vi "Close Active Workspace.vi"(8 "error in (no error)":errorcluster) -> (0 "error out":errorcluster)   [LabVIEW 2014]
uses:
  NationalInstruments.VeriStand.ClientAPI
  <vilib>/NI Veristand/Execution/Project/NI_VS Project ExecutionAPI.lvlib
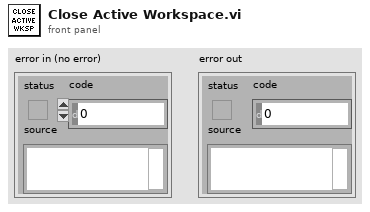
[diagram p1: front panel]
types:
  T1 = typedef "NI_VS Project ExecutionAPI.lvlib/Project Ref.ctl" = refnum<k24>
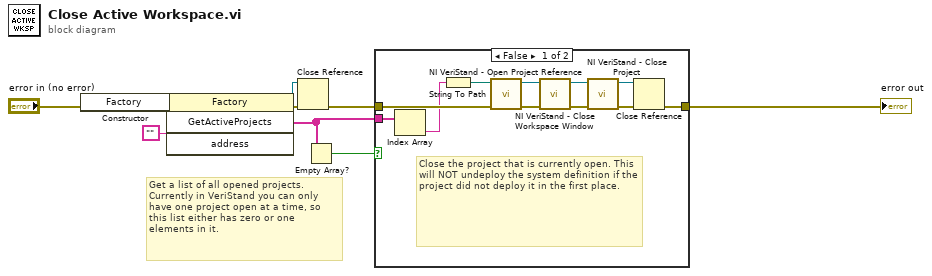
[diagram p0: block diagram]
diagram:
  # "Get a list of all opened projects. Currently in VeriStand you can only have one project open at a time, so this list either has zero or one elements in it."
  n1 = constructor class="Factory"(error in="error in (no error)") -> (reference out=w1:refnum<k24>, error out=w2:errorcluster)  [unwired: 2 in, 1 out]
  n2 = invoke class="Factory" method="GetActiveProjects"(reference=w1, error in=w2, "address"="") -> (reference out=w4:refnum<k24>, error out=w3:errorcluster, "GetActiveProjects"=w7:string[])  [unwired: 1 in, 1 out]
  n3 = Close Reference(reference=w4, error in (no error)=w3) -> (error out=w6:errorcluster)
  n4 = Empty Array?(array=w7) -> (empty?=w8:bool)
  n5 = case shown="False" w8 {
    tunnel: w7 -> [w21 _]
    tunnel: w6 -> [w20 w22]
    tunnel: [w15 w22] -> w9
    frame False {
      # "Close the project that is currently open. This will NOT undeploy the system definition if the project did not deploy it in the first place."
      n6 = Index Array(array=w21) -> (element=w19:string)  [unwired: 1 in]
      n7 = String To Path(string=w19) -> (path=w18:path)
      n8 = call <vilib>:"NI VeriStand - Open Project Reference.vi"("error in (no error)"=w20, "Project File Path"=w18) -> ("error out"=w13:errorcluster, "Project Ref"=w14:T1)  [unwired: 8 in]
      n9 = call <vilib>:"NI VeriStand - Close Workspace Window.vi"("error in (no error)"=w13, "Project Ref in"=w14) -> ("error out"=w12:errorcluster, "Project Ref out"=w11:T1)  [unwired: 8 in]
      n10 = call <vilib>:"NI VeriStand - Close Project.vi"("error in (no error)"=w12, "Project Ref in"=w11) -> ("error out"=w16:errorcluster, "Project Ref out"=w17:T1)  [unwired: 8 in]
      n11 = Close Reference(reference=w17, error in (no error)=w16) -> (error out=w15:errorcluster)
    }
    frame True {
      # "No project is open."
    }
  }
  "error out" <- w9
